vi "Data Sorting.vi"   [LabVIEW 2020]
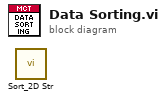
[diagram p0: block diagram]
diagram:
  n1 = call "Sort_2D Str.vi"() -> ()  [unwired: 10 in, 2 out]
